vi "CloseExternalDisplay-1.vi"(4 "error IN":errorcluster, 7 "[IN] # Window":i32) -> (0 "error OUT":errorcluster)   [LabVIEW 2020]
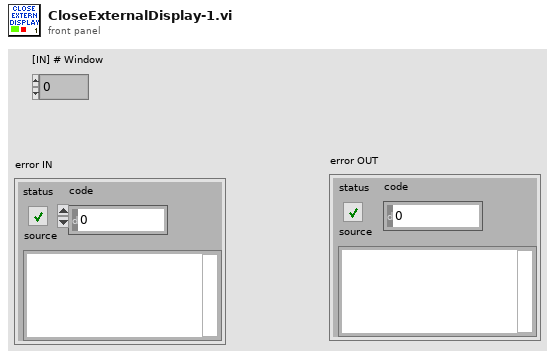
[diagram p1: front panel]
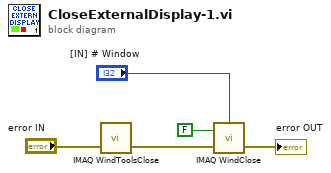
[diagram p0: block diagram]
diagram:
  n1 = call "IMAQ WindToolsClose"("error in (no error)"="error IN") -> ("error out"=w3:errorcluster)  [unwired: 5 in]
  n2 = call "IMAQ WindClose"("Window Number (0...15)"="[IN] # Window", "Close All Windows (False)"=FALSE, "error in (no error)"=w3) -> ("error out"=→"error OUT":errorcluster)  [unwired: 3 in]
